vi "ReadMarkers.vi"(10 "Data":string, 11 "Elements":i32=3) -> (1 "Remaining":string, 2 "Markers":sgl[][](array[numeric]), 3 "MarkerCount":u32)   [LabVIEW 2011]
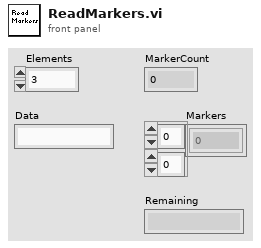
[diagram p1: front panel]
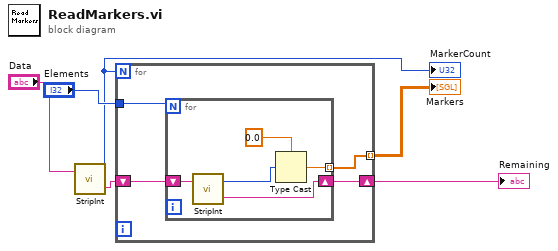
[diagram p0: block diagram]
diagram:
  n1 = call "StripInt.vi"("String"="Data") -> ("Remaining"=w3:string, "Value"=w4:u32)  [unwired: 1 in]
  "MarkerCount" <- w4
  n2 = for {
    N: w4 -> [_]
    shift-right: [w9] -> w2
    shift-left: w3 -> [w10]
    tunnel: [w8] -> w5 mode=indexing
    tunnel: "Elements" -> [w7]
    n3 = for {
      N: w7 -> [_]
      shift-right: [w14] -> w9
      shift-left: w10 -> [w15]
      tunnel: [w11] -> w8 mode=indexing
      n4 = call "StripInt.vi"("String"=w15) -> ("Remaining"=w14:string, "Value"=w13:u32)  [unwired: 1 in]
      n5 = Type Cast(type=sgl 0.0 ("single precision float"), x=w13) -> (*(type *) &x=w11:sgl)
    }
  }
  "Markers" <- w5
  "Remaining" <- w2
